vi "RSZVB Get Status Register.vi"(8 "error in (no error)":errorcluster {"code" format="%.0x"}, 10 "Status Registers Query (0: Operation Event)":i32(ring) items=["Operation Event", "Operation Condition", "Main Event", "Main Condition", "Limit Event Screen A", "Limit Condition Screen A", "Limit Event Screen B", "Limit Condition Screen B", "Integrity Event", "Integrity Condition", "Integrity Hardware Event", "Integrity Hardware Condition"], 11 "VISA session":refnum<visa-resource-name>) -> (0 "error out":errorcluster {"code" format="%.0x"}, 2 "Register Value":i32, 3 "dup VISA session":refnum<visa-resource-name>)   [LabVIEW 2011]
doc: "This VI contains the commands for the querying status reporting system.\n\nNote:\n\nFor detailed description of Status Reporting System see also operating manual.\n\nRemote-control command(s):\nSTATus:OPERation:EVENt?\nSTATus:OPERation:CONDition?\nSTATus:QUEStionable:EVENt?\nSTATus:QUEStionable:CONDition?\nSTATus:QUEStionable:LIMit<1|2>:EVENt?\nSTATus:QUEStionable:LIMit<1|2>:CONDition? \nSTATus:QUEStionable:INTegrity:EVENt?\nSTATus:QUEStionable:INTegrity:CONDition? \nSTATus:QUEStionable:INTegrity:HARDware:EVENt?\nSTATus:QUEStionable:INTegrity:HARDware:CONDition?"
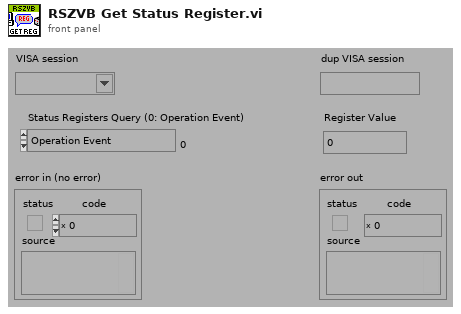
[diagram p1: front panel]
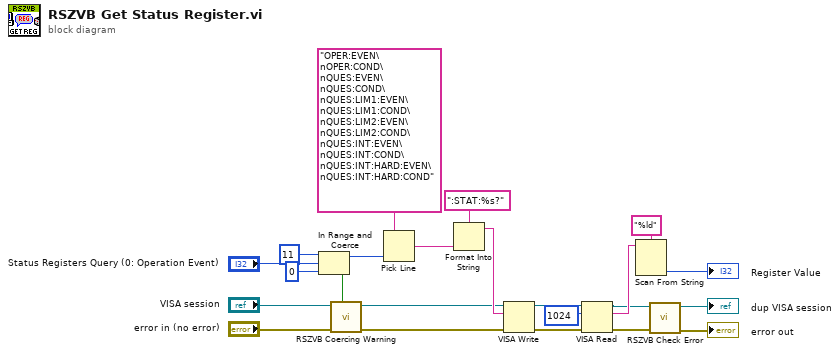
[diagram p0: block diagram]
diagram:
  n1 = In Range and Coerce(upper limit=11, x="Status Registers Query (0: Operation Event)", lower limit=0) -> (coerced(x)=w9:i32, In Range?=w14:bool)
  n2 = call "RSZVB Coercing Warning.vi"("In Range?"=w14, "error in (no error)"="error in (no error)", "VISA session"="VISA session") -> ("error out"=w18:errorcluster, "dup VISA session"=w17:refnum<visa-resource-name>)  [unwired: 7 in]
  n3 = Pick Line(multi-line string="OPER:EVEN\nOPER:COND\nQUES:EVEN\nQUES:COND\nQUES:LIM1:EVEN\nQUES:LIM1:COND\nQUES:LIM2:EVEN\nQUES:LIM2:COND\nQUES:INT:EVEN\nQUES:INT:COND\nQUES:INT:HARD:EVEN\nQUES:INT:HARD:COND", line index=w9) -> (output string=w10:string)  [unwired: 1 in]
  n4 = Format Into String(format string=":STAT:%s?", w10) -> (resulting string=w22:string)  [unwired: 2 in, 1 out]
  n5 = VISA Write(VISA resource name=w17, write buffer=w22, error in (no error)=w18) -> (VISA resource name out=w21:refnum<visa-resource-name>, error out=w20:errorcluster)  [unwired: 1 out]
  n6 = VISA Read(VISA resource name=w21, byte count=u32 1024 ("byte count (0)"), error in (no error)=w20) -> (VISA resource name out=w3:refnum<visa-resource-name>, read buffer=w13:string, error out=w2:errorcluster)  [unwired: 1 out]
  n7 = Scan From String(format string="%ld", input string=w13) -> (output 1=→"Register Value":i32)  [unwired: 3 in, 3 out]
  n8 = call "RSZVB Check Error.vi"("error in (no error)"=w2, "VISA session"=w3) -> ("error out"=→"error out":errorcluster, "dup VISA session"=→"dup VISA session":refnum<visa-resource-name>)  [unwired: 8 in]
